vi "configAutoSampling.vi"(5 "Port":u16, 7 "address":string, 8 "error in (no error)":errorcluster, 10 "Auto Sampling":bool, 11 "Instrument.Lockin in":refnum<class "Instrument.Lockin.lvclass">) -> (0 "error out":errorcluster, 3 "Instrument.Lockin out":refnum<class "Instrument.Lockin.lvclass">)   [LabVIEW 2016]
doc: "API to put lockin into IV mode.\n\nIf address=\"\", this API reads from localhost\nIf address is remote lockin, you need to add this computer to allowed whitelist on the lockin computer you are trying to access."
uses:
  Instrument.Lockin/Instrument.Lockin.lvclass
  Instrument.Lockin/Typedefs/Instrument.Lockin.Commands--Enum.ctl
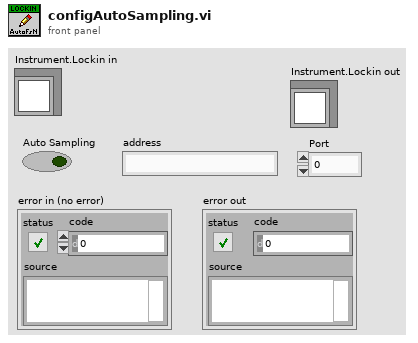
[diagram p1: front panel]
types:
  T1 = typedef "Instrument.Lockin.lvclass/Instrument.Lockin.Commands--Enum.ctl" = enum16{"configAO", "configAO_Amplitude", "configAO_DC", "configAO_Frequency", "configAO_Phase", "configAO_Function", "configAO_I+", "configREF", "configREF_Frequency", "configREF_Phase", "configREF_Filter", "configIVmode", "Reset", "configSampling", "Trigger", "getAO", "getAI", "getResults", "getTrigger", "getIVmode", "getSampling", "getAOconfig", "getREFconfig", "getREF_Filter", "configGain", "getGain", "configAutoSampling", "getAutoSampling"}
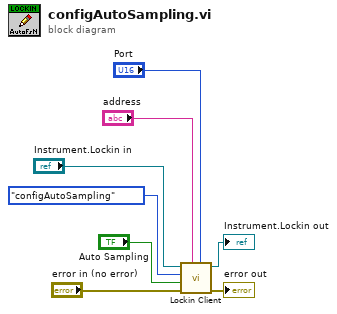
[diagram p0: block diagram]
diagram:
  n1 = call "Lockin Client.vi"("Port"="Port", "address"="address", "error in (no error)"="error in (no error)", "Data"="Auto Sampling", "Command"=Instrument.Lockin.Commands--Enum."configAutoSampling", "Instrument.Lockin in"="Instrument.Lockin in") -> ("error out"=→"error out":errorcluster, "Instrument.Lockin out"=→"Instrument.Lockin out":refnum<class "Instrument.Lockin.lvclass">)  [unwired: 3 in, 1 out]
